vi "microfono.vi"() -> ()   [LabVIEW 2011]
panel:
  in  "?":bool
  out "Data":dynamicdata(graph)
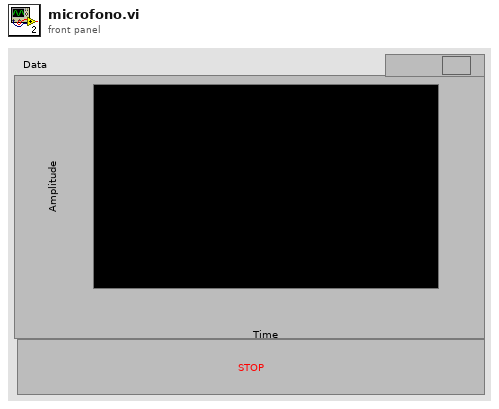
[diagram p1: front panel]
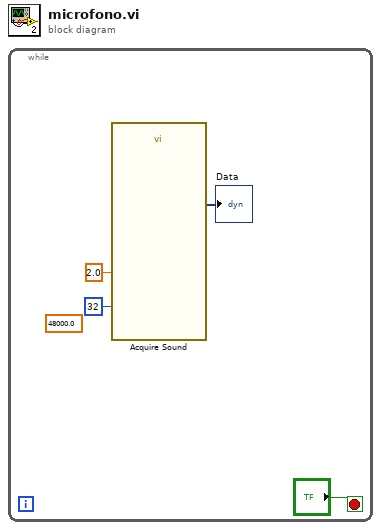
[diagram p0: block diagram]
diagram:
  n1 = while {
    stop <- "?" stop-if-true
    (unwired) 48000.0 ("Sample rate (Hz)")
    n2 = call "Acquire Sound"("Duration (s)"=2.0, "Resolution (bits)"=32) -> ("Data"=→"Data":dynamicdata)  [unwired: 16 in, 1 out]
  }
